vi "Find Next Section_Bool-Array-Cluster_.vi"(7 "Min Size":i32, 10 "Find":bool=TRUE, 11 "Array":cluster{"Array":bool[]}[](array[cluster])) -> (2 "Size Out":i32, 3 "Index Of Element Out":i32, 5 "Array Out":bool[](array[boolean]))   [LabVIEW 2024]
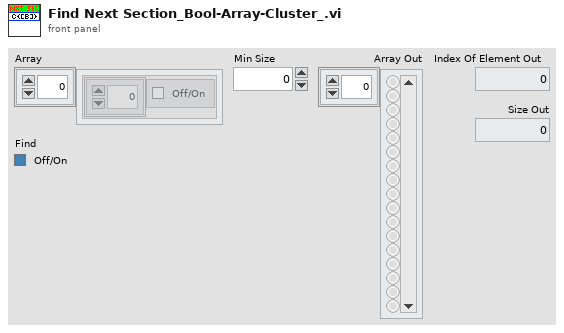
[diagram p1: front panel]
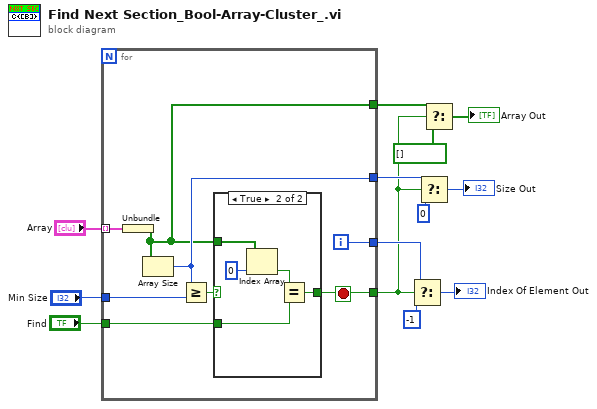
[diagram p0: block diagram]
diagram:
  n1 = for {
    tunnel: "Array" -> [w21] mode=indexing
    tunnel: "Min Size" -> [w20]
    tunnel: "Find" -> [w18]
    tunnel: [w17] -> w10
    tunnel: [w16] -> w3
    tunnel: [w15] -> w7
    tunnel: [w14] -> w4
    i -> [w17]
    stop <- w16 stop-if-true
    n2 = Unbundle(w21) -> ("Array"=w14:bool[])
    n3 = Array Size(array=w14) -> (size(s)=w15:i32)
    n4 = Greater Or Equal?(x=w15, y=w20) -> (x >= y?=w19:bool)
    n5 = case shown="True" w19 {
      selector: w19 -> [w22 _]
      tunnel: w14 -> [_ w27]
      tunnel: w18 -> [_ w24]
      tunnel: [w22 w23] -> w16
      frame False {
      }
      frame True {
        n6 = Index Array(array=w27, index=0) -> (element=w25:bool)
        n7 = Equal?(x=w25, y=w24) -> (x = y?=w23:bool)
      }
    }
  }
  n8 = Select(t=w10, s=w3, f=-1) -> (s? t:f=→"Index Of Element Out":i32)
  n9 = Select(t=w7, s=w3, f=0) -> (s? t:f=→"Size Out":i32)
  n10 = Select(t=w4, s=w3, f=bool[] []) -> (s? t:f=→"Array Out":bool[])
